vi "geradeaus weiter.vi"(8 "error in (no error)":errorcluster caption="Fehler (Eingang, kein Fehler)", 10 "fehlbearbeitung?":bool, 11 "Device ID":T1(ring)) -> (0 "error out":errorcluster caption="Fehler (Ausgang)", 3 "Device ID Out":T1(ring))   [LabVIEW 2010]
uses:
  globale Variable 1.vi
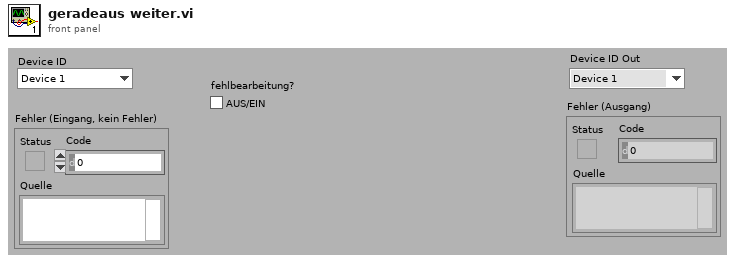
[diagram p1: front panel]
types:
  T1 = enum16{"Device 1", "Device 2", "Device 3", "Device 4", "Device 5", "Device 6", "Device 7", "Device 8"}
  T2 = enum8{"Robo Interface", "Extension 1", "Extension 2", "Extension 3"}
  T3 = enum8{"Output 1 (O1)", "Output 2 (O2)", "Output 3 (O3)", "Output 4 (O4)", "Output 5 (O5)", "Output 6 (O6)", "Output 7 (O7)", "Output 8 (O8)"}
  T4 = enum8{"Power 1", "Power 2", "Power 3", "Power 4", "Power 5", "Power 6", "Power 7", "Power 8"}
  T5 = enum8{"Goes High", "Goes Low", "Goes High or Low"}
  T6 = enum8{"Input 1 (I1)", "Input 2 (I2)", "Input 3 (I3)", "Input 4 (I4)", "Input 5 (I5)", "Input 6 (I6)", "Input 7 (I7)", "Input 8 (I8)"}
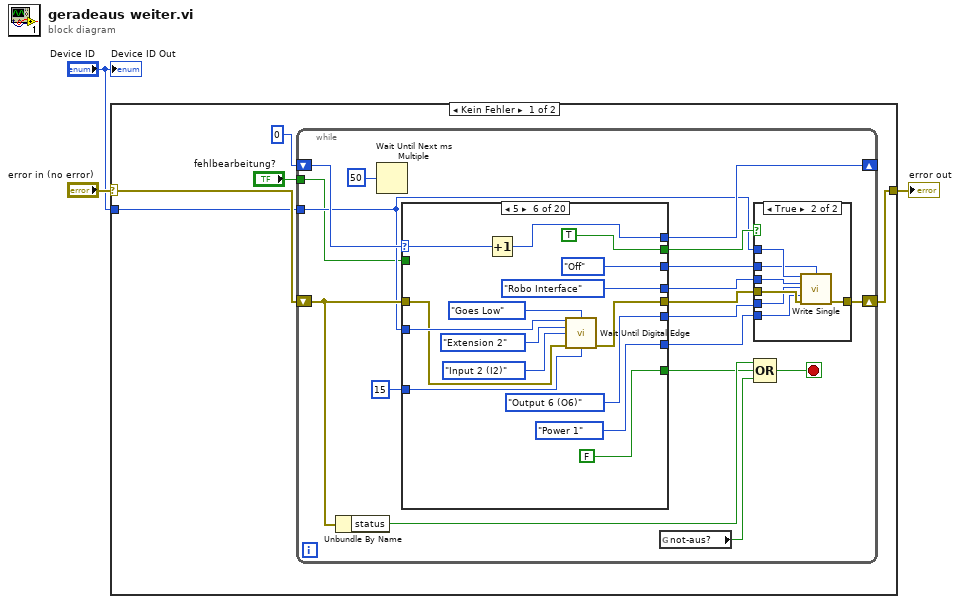
[diagram p0: block diagram]
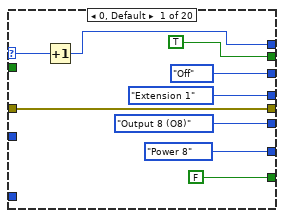
[diagram p3: hidden frame]
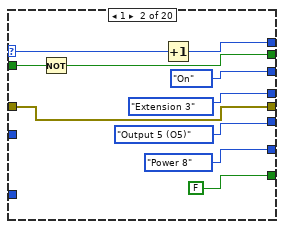
[diagram p4: hidden frame]
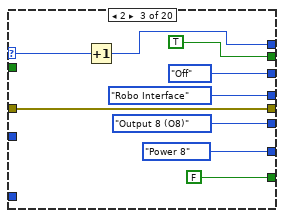
[diagram p5: hidden frame]
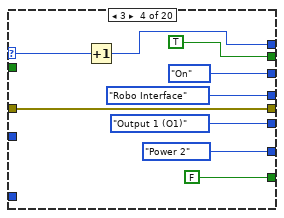
[diagram p6: hidden frame]
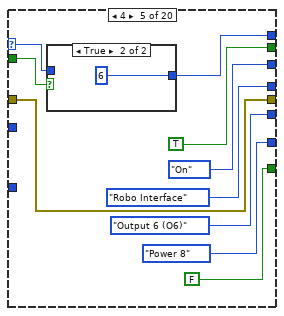
[diagram p7: hidden frame]
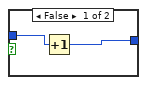
[diagram p8: hidden frame]
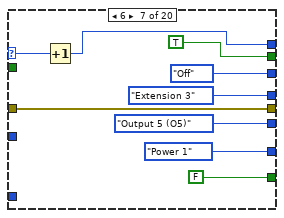
[diagram p9: hidden frame]
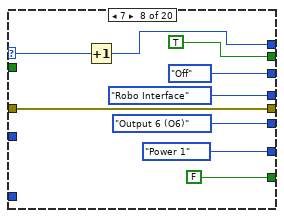
[diagram p10: hidden frame]
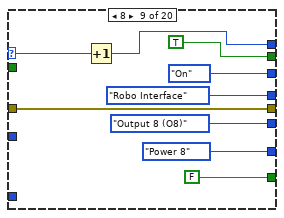
[diagram p11: hidden frame]
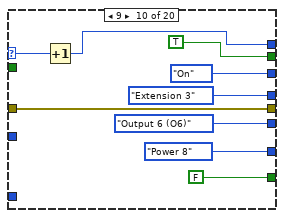
[diagram p12: hidden frame]
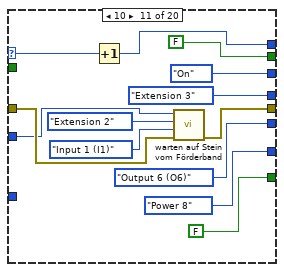
[diagram p13: hidden frame]
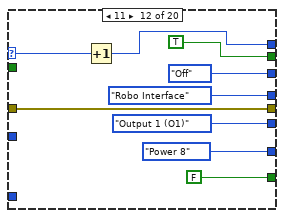
[diagram p14: hidden frame]
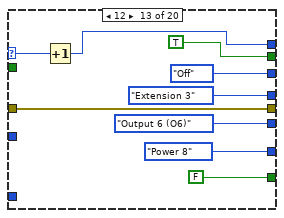
[diagram p15: hidden frame]
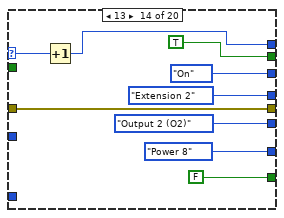
[diagram p16: hidden frame]
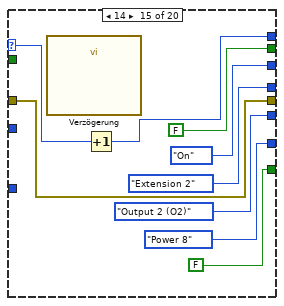
[diagram p17: hidden frame]
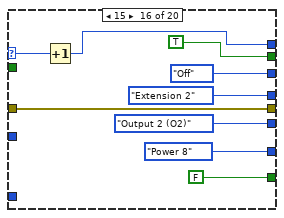
[diagram p18: hidden frame]
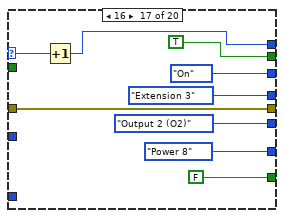
[diagram p19: hidden frame]
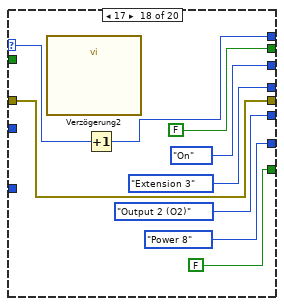
[diagram p20: hidden frame]
diagram:
  n1 = case shown="Kein Fehler" "error in (no error)" {
    selector: "error in (no error)" -> [w7 w229]
    tunnel: "Device ID" -> [w5 _]
    tunnel: [w6 w229] -> w1
    frame No Error {
      n2 = while {
        shift-right: [w24] -> _
        shift-left: 0 -> [w26]
        tunnel: w5 -> [w11]
        shift-right: [w20] -> w6
        shift-left: w7 -> [w19]
        tunnel: "fehlbearbeitung?" -> [w10]
        stop <- w22 stop-if-true
        n3 = Unbundle By Name(w19) -> ("status"=w23:bool)
        n4 = Wait Until Next ms Multiple(millisecond multiple=50) -> ()  [unwired: 1 out]
        n5 = case shown="5" w26 {
          selector: w26 -> [w42 w53 w61 w70 w80 w98 w107 w116 w125 w134 w147 w156 w165 w174 w183 w192 w201 w210 w219 w221]
          tunnel: [TRUE w44 TRUE TRUE TRUE TRUE TRUE TRUE TRUE TRUE FALSE TRUE TRUE TRUE FALSE TRUE TRUE FALSE TRUE FALSE] -> w25
          tunnel: [w41 w52 w60 w69 w79 w97 w106 w115 w124 w133 w146 w155 w164 w173 w182 w191 w200 w209 w218 w221] -> w24
          tunnel: [w40 w51 w59 w68 w78 w87 w100 w109 w118 w127 w136 w149 w158 w167 w176 w185 w194 w203 w212 w222] -> w21
          tunnel: w19 -> [w40 w51 w59 w68 w78 w88 w100 w109 w118 w127 w138 w149 w158 w167 w176 w185 w194 w203 w212 w222]
          tunnel: [T2."Extension 1" ("Module") T2."Extension 3" ("Module") T2."Robo Interface" ("Module") T2."Robo Interface" ("Module") T2."Robo Interface" ("Module") T2."Robo Interface" ("Module") T2."Extension 3" ("Module") T2."Robo Interface" ("Module") T2."Robo Interface" ("Module") T2."Extension 3" ("Module") T2."Extension 3" ("Module") T2."Robo Interface" ("Module") T2."Extension 3" ("Module") T2."Extension 2" ("Module") T2."Extension 2" ("Module") T2."Extension 2" ("Module") T2."Extension 3" ("Module") T2."Extension 3" ("Module") T2."Extension 3" ("Module") T2."Extension 3" ("Module")] -> w18
          tunnel: [T3."Output 8 (O8)" ("Single_Output") T3."Output 5 (O5)" ("Single_Output") T3."Output 8 (O8)" ("Single_Output") T3."Output 1 (O1)" ("Single_Output") T3."Output 6 (O6)" ("Single_Output") T3."Output 6 (O6)" ("Single_Output") T3."Output 5 (O5)" ("Single_Output") T3."Output 6 (O6)" ("Single_Output") T3."Output 8 (O8)" ("Single_Output") T3."Output 6 (O6)" ("Single_Output") T3."Output 6 (O6)" ("Single_Output") T3."Output 1 (O1)" ("Single_Output") T3."Output 6 (O6)" ("Single_Output") T3."Output 2 (O2)" ("Single_Output") T3."Output 2 (O2)" ("Single_Output") T3."Output 2 (O2)" ("Single_Output") T3."Output 2 (O2)" ("Single_Output") T3."Output 2 (O2)" ("Single_Output") T3."Output 2 (O2)" ("Single_Output") T3."Output 2 (O2)" ("Single_Output")] -> w17
          tunnel: [T4."Power 8" ("Output_PWM") T4."Power 8" ("Output_PWM") T4."Power 8" ("Output_PWM") T4."Power 2" ("Output_PWM") T4."Power 8" ("Output_PWM") T4."Power 1" ("Output_PWM") T4."Power 1" ("Output_PWM") T4."Power 1" ("Output_PWM") T4."Power 8" ("Output_PWM") T4."Power 8" ("Output_PWM") T4."Power 8" ("Output_PWM") T4."Power 8" ("Output_PWM") T4."Power 8" ("Output_PWM") T4."Power 8" ("Output_PWM") T4."Power 8" ("Output_PWM") T4."Power 8" ("Output_PWM") T4."Power 8" ("Output_PWM") T4."Power 8" ("Output_PWM") T4."Power 8" ("Output_PWM") T4."Power 8" ("Output_PWM")] -> w16
          tunnel: [enum8{"Off", "On"}."Off" ("Output_Action") enum8{"Off", "On"}."On" ("Output_Action") enum8{"Off", "On"}."Off" ("Output_Action") enum8{"Off", "On"}."On" ("Output_Action") enum8{"Off", "On"}."On" ("Output_Action") enum8{"Off", "On"}."Off" ("Output_Action") enum8{"Off", "On"}."Off" ("Output_Action") enum8{"Off", "On"}."Off" ("Output_Action") enum8{"Off", "On"}."On" ("Output_Action") enum8{"Off", "On"}."On" ("Output_Action") enum8{"Off", "On"}."On" ("Output_Action") enum8{"Off", "On"}."Off" ("Output_Action") enum8{"Off", "On"}."Off" ("Output_Action") enum8{"Off", "On"}."On" ("Output_Action") enum8{"Off", "On"}."On" ("Output_Action") enum8{"Off", "On"}."Off" ("Output_Action") enum8{"Off", "On"}."On" ("Output_Action") enum8{"Off", "On"}."On" ("Output_Action") enum8{"Off", "On"}."Off" ("Output_Action") enum8{"Off", "On"}."Off" ("Output_Action")] -> w15
          tunnel: [FALSE FALSE FALSE FALSE FALSE FALSE FALSE FALSE FALSE FALSE FALSE FALSE FALSE FALSE FALSE FALSE FALSE FALSE FALSE TRUE] -> w12
          tunnel: w11 -> [_ _ _ _ _ w91 _ _ _ _ w137 _ _ _ _ _ _ _ _ _]
          tunnel: w10 -> [_ w45 _ _ w72 _ _ _ _ _ _ _ _ _ _ _ _ _ _ _]
          tunnel: 15 -> [_ _ _ _ _ w85 _ _ _ _ _ _ _ _ _ _ _ _ _ _]
          frame 0, Default {
            n6 = Increment(x=w42) -> (x+1=w41:i32)
          }
          frame 1 {
            n7 = Not(x=w45) -> (.not. x?=w44:bool)
            n8 = Increment(x=w53) -> (x+1=w52:i32)
          }
          frame 2 {
            n9 = Increment(x=w61) -> (x+1=w60:i32)
          }
          frame 3 {
            n10 = Increment(x=w70) -> (x+1=w69:i32)
          }
          frame 4 {
            n11 = case shown="TRUE" w72 {
              tunnel: w80 -> [w83 _]
              tunnel: [w82 6] -> w79
              frame False {
                n12 = Increment(x=w83) -> (x+1=w82:i32)
              }
              frame True {
              }
            }
          }
          frame 5 {
            n13 = Increment(x=w98) -> (x+1=w97:i32)
            n14 = call "Wait Until Digital Edge.vi"("Device ID"=w91, "Wait Until"=T5."Goes Low", "Module"=T2."Extension 2", "Digital_Input"=T6."Input 2 (I2)", "error in"=w88, "Time Out (10)"=w85) -> ("error out"=w87:errorcluster)  [unwired: 9 out]
          }
          frame 6 {
            n15 = Increment(x=w107) -> (x+1=w106:i32)
          }
          frame 7 {
            n16 = Increment(x=w116) -> (x+1=w115:i32)
          }
          frame 8 {
            n17 = Increment(x=w125) -> (x+1=w124:i32)
          }
          frame 9 {
            n18 = Increment(x=w134) -> (x+1=w133:i32)
          }
          frame 10 {
            n19 = Increment(x=w147) -> (x+1=w146:i32)
            n20 = call "warten auf Stein vom Förderband.vi"("error in (no error)"=w138, "Digital_Input"=T6."Input 1 (I1)", "Module"=T2."Extension 2", "Device ID"=w137) -> ("error out"=w136:errorcluster)  [unwired: 7 out]
          }
          frame 11 {
            n21 = Increment(x=w156) -> (x+1=w155:i32)
          }
          frame 12 {
            n22 = Increment(x=w165) -> (x+1=w164:i32)
          }
          frame 13 {
            n23 = Increment(x=w174) -> (x+1=w173:i32)
          }
          frame 14 {
            n24 = call "Verzögerung"() -> ()  [unwired: 2 in, 10 out]
            n25 = Increment(x=w183) -> (x+1=w182:i32)
          }
          frame 15 {
            n26 = Increment(x=w192) -> (x+1=w191:i32)
          }
          frame 16 {
            n27 = Increment(x=w201) -> (x+1=w200:i32)
          }
          frame 17 {
            n28 = call "Verzögerung2"() -> ()  [unwired: 2 in, 10 out]
            n29 = Increment(x=w210) -> (x+1=w209:i32)
          }
          frame 18 {
            n30 = Increment(x=w219) -> (x+1=w218:i32)
          }
          frame 19 {
          }
        }
        n31 = global read "globale Variable 1.vi" "not-aus?"() -> (w13:bool)
        n32 = case shown="TRUE" w25 {
          tunnel: w11 -> [_ w34]
          tunnel: w21 -> [w27 w33]
          tunnel: [w27 w32] -> w20
          tunnel: w18 -> [_ w31]
          tunnel: w17 -> [_ w30]
          tunnel: w16 -> [_ w29]
          tunnel: w15 -> [_ w28]
          frame False {
          }
          frame True {
            n33 = call "Write Single.vi"("Device ID"=w34, "Output_Action"=w28, "Module"=w31, "Single_Output"=w30, "Output_PWM"=w29, "error in"=w33) -> ("error out"=w32:errorcluster)  [unwired: 9 out]
          }
        }
        n34 = Compound Arithmetic op=OR(w23, w12, w13) -> (w22:bool)
      }
    }
    frame Error {
    }
  }
  "error out" <- w1
  "Device ID Out" <- "Device ID"
